vi "table 2.vi"() -> ()   [LabVIEW 2020]
panel:
  out "Array":dbl[][](array[numeric])
  in  "end number":dbl
  in  "start number":dbl
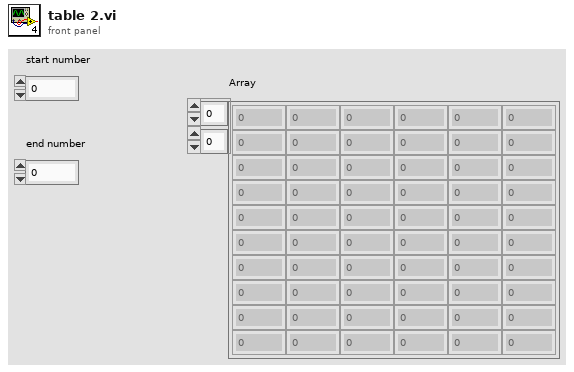
[diagram p1: front panel]
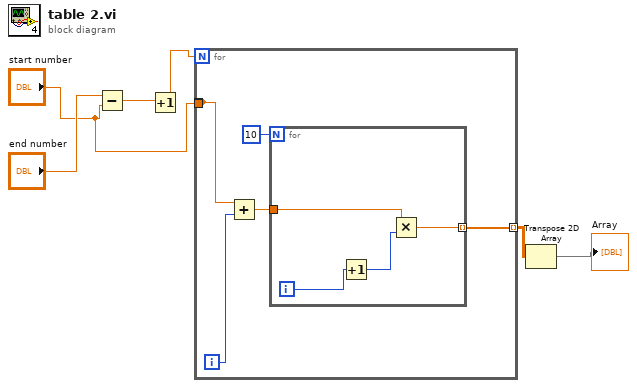
[diagram p0: block diagram]
diagram:
  n1 = Subtract(x="end number", y="start number") -> (x-y=w6:dbl)
  n2 = Increment(x=w6) -> (x+1=w5:dbl)
  n3 = for {
    N: w5 -> [_]
    tunnel: [w11] -> _ mode=indexing
    tunnel: "start number" -> [w11]
    tunnel: [w7] -> w2 mode=indexing
    i -> [w8]
    n4 = Add(x=w11, y=w8) -> (x+y=w9:dbl)
    n5 = for {
      N: 10 -> [_]
      tunnel: w9 -> [w13]
      tunnel: [w12] -> w7 mode=indexing
      i -> [w15]
      n6 = Increment(x=w15) -> (x+1=w14:i32)
      n7 = Multiply(x=w13, y=w14) -> (x*y=w12:dbl)
    }
  }
  n8 = Transpose 2D Array(2D array=w2) -> (transposed array=→"Array":dbl[][])
